vi "test_read-nmea-data2.vi"() -> ()   [LabVIEW 2019] (continued)
23,06,64,050,35,6*6E\n\t\n15:13:22.46\tF9P\t$GPGSV,3,2,09,09,45,074,31,12,23,276,26,17,33,154,28,19,52,157,,6*67\n\t\n15:13:22.48\tF9P\t$GPGSV,3,3,09,25,12,306,,6*5B\n\t\n15:13:22.50\tF9P\t$GLGSV,2,1,08,69,11,031,36,70,70,038,25,71,53,206,41,72,05,210,19,1*7D\n\t\n15:13:22.52\tF9P\t$GLGSV,2,2,08,77,01,325,,84,19,123,11,85,70,070,32,86,37,330,,1*77\n\t\n15:13:22.54\tF9P\t$GLGSV,2,1,08,69,11,031,26,70,70,038,,71,53,206,27,72,05,210,,3*71\n\t\n15:13:22.56\tF9P\t$GLGSV,2,2,08,77,01,325,,84,19,123,17,85,70,070,24,86,37,330,,3*74\n\t\n15:13:22.58\tF9P\t$GAGSV,2,1,08,02,08,297,11,04,66,116,30,09,32,193,35,11,72,359,26,7*74\n\t\n15:13:22.60\tF9P\t$GAGSV,2,2,08,12,40,103,32,19,26,045,18,25,09,249,,36,26,308,21,7*73\n\t\n15:13:22.62\tF9P\t$GAGSV,2,1,08,02,08,297,,04,66,116,,09,32,193,,11,72,359,,2*70\n\t\n15:13:22.64\tF9P\t$GAGSV,2,2,08,12,40,103,,19,26,045,,25,09,249,,36,26,308,,2*7D\n\t\n15:13:22.66\tF9P\t$GBGSV,1,1,04,11,49,132,29,14,87,114,27,28,,,29,33,61,220,32,1*48\n\t\n15:13:22.68\tF9P\t$GBGSV,1,1,04,11,49,132,34,14,87,114,,25,,,05,33,61,220,,3*41\n\t\n15:13:22.70\tF9P\t$GNGLL,3723.55902,N,12656.98306,E,061324.00,A,A*79\n\t\n15:13:22.72\tF9P\t\t\n15:13:22.74\tF9P\t\t\n15:13:22.76\tF9P\t\t\n15:13:22.78\tF9P\t\t\n15:13:22.80\tF9P\t\t\n15:13:22.82\tF9P\t\t\n15:13:22.84\tF9P\t\t\n15:13:22.86\tF9P\t\t\n15:13:22.88\tF9P\t\t\n15:13:22.90\tF9P\t\t\n15:13:22.92\tF9P\t\t\n15:13:22.94\tF9P\t\t\n15:13:22.96\tF9P\t\t\n15:13:22.98\tF9P\t\t\n15:13:23.00\tF9P\t\t\n15:13:23.02\tF9P\t\t\n15:13:23.04\tF9P\t\t\n15:13:23.06\tF9P\t\t\n15:13:23.08\tF9P\t\t\n15:13:23.10\tF9P\t\t\n15:13:23.12\tF9P\t\t\n15:13:23.14\tF9P\t\t\n15:13:23.16\tF9P\t\t\n15:13:23.18\tF9P\t\t\n15:13:23.20\tF9P\t\t\n15:13:23.22\tF9P\t\t\n15:13:23.24\tF9P\t$GNRMC,061325.00,A,3723.55967,N,12656.98378,E,2.656,30.39,250720,,,A,V*33\n\t\n15:13:23.26\tF9P\t$GNVTG,30.39,T,,M,2.656,N,4.919,K,A*18\n\t\n15:13:23.28\tF9P\t$GNGGA,061325.00,3723.55967,N,12656.98378,E,1,12,0.68,50.1,M,18.5,M,,*72\n\t\n15:13:23.30\tF9P\t$GNGSA,A,3,12,06,19,05,17,09,04,02,,,,,1.20,0.68,0.99,1*0D\n\t\n15:13:23.32\tF9P\t$GNGSA,A,3,85,70,71,84,,,,,,,,,1.20,0.68,0.99,2*0F\n\t\n15:13:23.34\tF9P\t$GNGSA,A,3,36,19,11,04,09,12,,,,,,,1.20,0.68,0.99,3*0D\n\t\n15:13:23.36\tF9P\t$GNGSA,A,3,14,11,33,,,,,,,,,,1.20,0.68,0.99,4*0C\n\t\n15:13:23.38\tF9P\t$GPGSV,3,1,09,02,55,320,30,04,17,043,23,05,38,248,37,06,64,050,30,1*6D\n\t\n15:13:23.40\tF9P\t$GPGSV,3,2,09,09,45,074,33,12,23,276,39,17,33,154,37,19,52,157,31,1*60\n\t\n15:13:23.42\tF9P\t$GPGSV,3,3,09,25,12,306,21,1*5F\n\t\n15:13:23.44\tF9P\t$GPGSV,3,1,09,02,55,320,,04,17,043,16,05,38,248,22,06,64,050,35,6*6E\n\t\n15:13:23.46\tF9P\t$GPGSV,3,2,09,09,45,074,33,12,23,276,26,17,33,154,27,19,52,157,,6*6A\n\t\n15:13:23.48\tF9P\t$GPGSV,3,3,09,25,12,306,,6*5B\n\t\n15:13:23.50\tF9P\t$GLGSV,2,1,08,69,11,031,31,70,70,038,25,71,53,206,33,72,05,210,21,1*74\n\t\n15:13:23.52\tF9P\t$GLGSV,2,2,08,77,01,325,,84,19,123,14,85,70,070,39,86,37,330,,1*79\n\t\n15:13:23.54\tF9P\t$GLGSV,2,1,08,69,11,031,31,70,70,038,,71,53,206,25,72,05,210,,3*75\n\t\n15:13:23.56\tF9P\t$GLGSV,2,2,08,77,01,325,,84,19,123,16,85,70,070,25,86,37,330,,3*74\n\t\n15:13:23.58\tF9P\t$GAGSV,2,1,08,02,08,297,08,04,66,116,29,09,32,193,37,11,72,359,27,7*77\n\t\n15:13:23.60\tF9P\t$GAGSV,2,2,08,12,40,103,27,19,26,045,18,25,09,249,,36,26,308,20,7*76\n\t\n15:13:23.62\tF9P\t$GAGSV,2,1,08,02,08,297,,04,66,116,,09,32,193,,11,72,359,,2*70\n\t\n15:13:23.64\tF9P\t$GAGSV,2,2,08,12,40,103,,19,26,045,,25,09,249,,36,26,308,,2*7D\n\t\n15:13:23.66\tF9P\t$GBGSV,1,1,04,11,49,132,33,14,87,114,28,28,,,29,33,61,220,27,1*48\n\t\n15:13:23.68\tF9P\t$GBGSV,1,1,03,11,49,132,30,14,87,114,,33,61,220,,3*40\n\t\n15:13:23.70\tF9P\t$GNGLL,3723.55967,N,12656.98378,E,061325.00,A,A*72\n\t\n15:13:23.72\tF9P\t\t\n15:13:23.74\tF9P\t\t\n15:13:23.76\tF9P\t\t\n15:13:23.78\tF9P\t\t\n15:13:23.80\tF9P\t\t\n15:13:23.82\tF9P\t\t\n15:13:23.84\tF9P\t\t\n15:13:23.86\tF9P\t\t\n15:13:23.88\tF9P\t\t\n15:13:23.90\tF9P\t\t\n15:13:23.92\tF9P\t\t\n15:13:23.94\tF9P\t\t\n15:13:23.96\tF9P\t\t\n15:13:23.98\tF9P\t\t\n15:13:24.00\tF9P\t\t\n15:13:24.02\tF9P\t\t\n15:13:24.04\tF9P\t\t\n15:13:24.06\tF9P\t\t\n15:13:24.08\tF9P\t\t\n15:13:24.10\tF9P\t\t\n15:13:24.12\tF9P\t\t\n15:13:24.14\tF9P\t\t\n15:13:24.16\tF9P\t\t\n15:13:24.18\tF9P\t\t\n15:13:24.20\tF9P\t\t\n15:13:24.22\tF9P\t\t\n15:13:24.24\tF9P\t$GNRMC,061326.00,A,3723.56015,N,12656.98454,E,2.542,31.14,250720,,,A,V*3E\n\t\n15:13:24.26\tF9P\t$GNVTG,31.14,T,,M,2.542,N,4.708,K,A*1E\n\t\n15:13:24.28\tF9P\t$GNGGA,061326.00,3723.56015,N,12656.98454,E,1,12,0.71,50.6,M,18.5,M,,*78\n\t\n15:13:24.30\tF9P\t$GNGSA,A,3,12,06,19,05,17,09,04,02,,,,,1.26,0.71,1.04,1*06\n\t\n15:13:24.32\tF9P\t$GNGSA,A,3,85,70,71,84,,,,,,,,,1.26,0.71,1.04,2*04\n\t\n15:13:24.34\tF9P\t$GNGSA,A,3,36,19,11,04,09,12,,,,,,,1.26,0.71,1.04,3*06\n\t\n15:13:24.36\tF9P\t$GNGSA,A,3,14,11,33,,,,,,,,,,1.26,0.71,1.04,4*07\n\t\n15:13:24.38\tF9P\t$GPGSV,3,1,09,02,55,320,35,04,17,043,23,05,38,248,26,06,64,050,30,1*68\n\t\n15:13:24.40\tF9P\t$GPGSV,3,2,09,09,45,074,36,12,23,276,42,17,33,154,30,19,52,157,29,1*67\n\t\n15:13:24.42\tF9P\t$GPGSV,3,3,09,25,12,306,20,1*5E\n\t\n15:13:24.44\tF9P\t$GPGSV,3,1,09,02,55,320,,04,17,043,15,05,38,248,18,06,64,050,31,6*60\n\t\n15:13:24.46\tF9P\t$GPGSV,3,2,09,09,45,074,33,12,23,276,26,17,33,154,24,19,52,157,,6*69\n\t\n15:13:24.48\tF9P\t$GPGSV,3,3,09,25,12,306,,6*5B\n\t\n15:13:24.50\tF9P\t$GLGSV,2,1,08,69,11,031,33,70,70,038,26,71,53,206,33,72,05,210,21,1*75\n\t\n15:13:24.52\tF9P\t$GLGSV,2,2,08,77,01,325,,84,19,123,08,85,70,070,31,86,37,330,,1*7C\n\t\n15:13:24.54\tF9P\t$GLGSV,2,1,08,69,11,031,31,70,70,038,,71,53,206,24,72,05,210,,3*74\n\t\n15:13:24.56\tF9P\t$GLGSV,2,2,08,77,01,325,,84,19,123,16,85,70,070,27,86,37,330,,3*76\n\t\n15:13:24.58\tF9P\t$GAGSV,2,1,08,02,08,297,11,04,66,116,33,09,32,193,39,11,72,359,27,7*7A\n\t\n15:13:24.60\tF9P\t$GAGSV,2,2,08,12,40,103,32,19,26,045,18,25,09,249,,36,26,308,21,7*73\n\t\n15:13:24.62\tF9P\t$GAGSV,2,1,08,02,08,297,,04,66,116,,09,32,193,,11,72,359,,2*70\n\t\n15:13:24.64\tF9P\t$GAGSV,2,2,08,12,40,103,,19,26,045,,25,09,249,,36,26,308,,2*7D\n\t\n15:13:24.66\tF9P\t$GBGSV,1,1,04,11,49,132,27,14,87,114,33,28,,,33,33,61,220,32,1*48\n\t\n15:13:24.68\tF9P\t$GBGSV,1,1,03,11,49,132,29,14,87,114,,33,61,220,,3*48\n\t\n15:13:24.70\tF9P\t$GNGLL,3723.56015,N,12656.98454,E,061326.00,A,A*77\n\t\n15:13:24.72\tF9P\t\t\n15:13:24.74\tF9P\t\t\n15:13:24.76\tF9P\t\t\n15:13:24.78\tF9P\t\t\n15:13:24.80\tF9P\t\t\n15:13:24.82\tF9P\t\t\n15:13:24.84\tF9P\t\t\n15:13:24.86\tF9P\t\t\n15:13:24.88\tF9P\t\t\n15:13:24.90\tF9P\t\t\n15:13:24.92\tF9P\t\t\n15:13:24.94\tF9P\t\t\n15:13:24.96\tF9P\t\t\n15:13:24.98\tF9P\t\t\n15:13:25.00\tF9P\t\t\n15:13:25.02\tF9P\t\t\n15:13:25.04\tF9P\t\t\n15:13:25.06\tF9P\t\t\n15:13:25.08\tF9P\t\t\n15:13:25.10\tF9P\t\t\n15:13:25.12\tF9P\t\t\n15:13:25.14\tF9P\t\t\n15:13:25.16\tF9P\t\t\n15:13:25.18\tF9P\t\t\n15:13:25.20\tF9P\t\t\n15:13:25.22\tF9P\t\t\n15:13:25.24\tF9P\t$GNRMC,061327.00,A,3723.56072,N,12656.98531,E,2.555,25.42,250720,,,A,V*3C\n\t\n15:13:25.26\tF9P\t$GNVTG,25.42,T,,M,2.555,N,4.733,K,A*16\n\t\n15:13:25.28\tF9P\t$GNGGA,061327.00,3723.56072,N,12656.98531,E,1,12,0.71,50.7,M,18.5,M,,*7B\n\t\n15:13:25.30\tF9P\t$GNGSA,A,3,12,06,19,05,17,09,04,02,,,,,1.26,0.71,1.04,1*06\n\t\n15:13:25.32\tF9P\t$GNGSA,A,3,85,70,71,84,,,,,,,,,1.26,0.71,1.04,2*04\n\t\n15:13:25.34\tF9P\t$GNGSA,A,3,36,19,11,04,09,12,,,,,,,1.26,0.71,1.04,3*06\n\t\n15:13:25.36\tF9P\t$GNGSA,A,3,14,11,33,,,,,,,,,,1.26,0.71,1.04,4*07\n\t\n15:13:25.38\tF9P\t$GPGSV,3,1,09,02,55,320,28,04,17,043,24,05,38,248,40,06,64,050,33,1*60\n\t\n15:13:25.40\tF9P\t$GPGSV,3,2,09,09,44,073,28,12,23,276,46,17,33,154,38,19,52,157,31,1*6B\n\t\n15:13:25.42\tF9P\t$GPGSV,3,3,09,25,12,306,19,1*54\n\t\n15:13:25.44\tF9P\t$GPGSV,3,1,09,02,55,320,,04,17,043,15,05,38,248,17,06,64,050,32,6*6C\n\t\n15:13:25.46\tF9P\t$GPGSV,3,2,09,09,44,073,35,12,23,276,25,17,33,154,25,19,52,157,,6*6B\n\t\n15:13:25.48\tF9P\t$GPGSV,3,3,09,25,12,306,,6*5B\n\t\n15:13:25.50\tF9P\t$GLGSV,2,1,08,69,11,031,33,70,70,038,26,71,53,206,34,72,05,210,20,1*73\n\t\n15:13:25.52\tF9P\t$GLGSV,2,2,08,77,01,325,,84,19,123,11,85,70,070,32,86,37,330,,1*77\n\t\n15:13:25.54\tF9P\t$GLGSV,2,1,08,69,11,031,23,70,70,038,,71,53,206,25,72,05,210,,3*76\n\t\n15:13:25.56\tF9P\t$GLGSV,2,2,08,77,01,325,,84,19,123,18,85,70,070,26,86,37,330,,3*79\n\t\n15:13:25.58\tF9P\t$GAGSV,2,1,08,02,08,297,10,04,66,116,28,09,32,193,38,11,72,359,27,7*70\n\t\n15:13:25.60\tF9P\t$GAGSV,2,2,08,12,40,103,28,19,26,045,17,25,09,249,,36,26,308,20,7*76\n\t\n15:13:25.62\tF9P\t$GAGSV,2,1,08,02,08,297,,04,66,116,,09,32,193,,11,72,359,,2*70\n\t\n15:13:25.64\tF9P\t$GAGSV,2,2,08,12,40,103,,19,26,045,,25,09,249,,36,26,308,,2*7D\n\t\n15:13:25.66\tF9P\t$GBGSV,1,1,04,11,49,132,28,14,87,114,31,28,,,32,33,61,220,28,1*4F\n\t\n15:13:25.68\tF9P\t$GBGSV,1,1,03,11,49,132,32,14,87,114,,33,61,220,,3*42\n\t\n15:13:25.70\tF9P\t$GNGLL,3723.56072,N,12656.98531,E,061327.00,A,A*75\n\t\n15:13:25.72\tF9P\t\t\n15:13:25.74\tF9P\t\t\n15:13:25.76\tF9P\t\t\n15:13:25.78\tF9P\t\t\n15:13:25.80\tF9P\t\t\n15:13:25.82\tF9P\t\t\n15:13:25.84\tF9P\t\t\n15:13:25.86\tF9P\t\t\n15:13:25.88\tF9P\t\t\n15:13:25.90\tF9P\t\t\n15:13:25.92\tF9P\t\t\n15:13:25.94\tF9P\t\t\n15:13:25.96\tF9P\t\t\n15:13:25.98\tF9P\t\t\n15:13:26.00\tF9P\t\t\n15:13:26.02\tF9P\t\t\n15:13:26.04\tF9P\t\t\n15:13:26.06\tF9P\t\t\n15:13:26.08\tF9P\t\t\n15:13:26.10\tF9P\t\t\n15:13:26.12\tF9P\t\t\n15:13:26.14\tF9P\t\t\n15:13:26.16\tF9P\t\t\n15:13:26.18\tF9P\t\t\n15:13:26.20\tF9P\t\t\n15:13:26.22\tF9P\t\t\n15:13:26.24\tF9P\t$GNRMC,061328.00,A,3723.56131,N,12656.98590,E,2.306,24.51,250720,,,A,V*3D\n\t\n15:13:26.26\tF9P\t$GNVTG,24.51,T,,M,2.306,N,4.270,K,A*17\n\t\n15:13:26.28\tF9P\t$GNGGA,061328.00,3723.56131,N,12656.98590,E,1,12,0.84,50.2,M,18.5,M,,*76\n\t\n15:13:26.30\tF9P\t$GNGSA,A,3,12,06,19,05,17,09,04,02,,,,,1.55,0.84,1.30,1*0F\n\t\n15:13:26.32\tF9P\t$GNGSA,A,3,85,70,71,84,,,,,,,,,1.55,0.84,1.30,2*0D\n\t\n15:13:26.34\tF9P\t$GNGSA,A,3,36,19,11,04,09,12,,,,,,,1.55,0.84,1.30,3*0F\n\t\n15:13:26.36\tF9P\t$GNGSA,A,3,14,11,33,,,,,,,,,,1.55,0.84,1.30,4*0E\n\t\n15:13:26.38\tF9P\t$GPGSV,3,1,09,02,55,320,32,04,17,043,22,05,38,248,34,06,64,050,30,1*6D\n\t\n15:13:26.40\tF9P\t$GPGSV,3,2,09,09,44,073,28,12,23,276,48,17,33,154,42,19,52,157,28,1*60\n\t\n15:13:26.42\tF9P\t$GPGSV,3,3,09,25,12,306,20,1*5E\n\t\n15:13:26.44\tF9P\t$GPGSV,3,1,09,02,55,320,,04,17,043,16,05,38,248,20,06,64,050,31,6*68\n\t\n15:13:26.46\tF9P\t$GPGSV,3,2,09,09,44,073,35,12,23,276,24,17,33,154,28,19,52,157,,6*67\n\t\n15:13:26.48\tF9P\t$GPGSV,3,3,09,25,12,306,,6*5B\n\t\n15:13:26.50\tF9P\t$GLGSV,2,1,08,69,11,031,33,70,70,038,23,71,53,206,39,72,05,210,20,1*7B\n\t\n15:13:26.52\tF9P\t$GLGSV,2,2,08,77,01,325,,84,19,123,17,85,70,070,32,86,37,330,,1*71\n\t\n15:13:26.54\tF9P\t$GLGSV,2,1,08,69,11,031,25,70,70,038,,71,53,206,26,72,05,210,,3*73\n\t\n15:13:26.56\tF9P\t$GLGSV,2,2,08,77,01,325,,84,19,123,20,85,70,070,25,86,37,330,,3*71\n\t\n15:13:26.58\tF9P\t$GAGSV,2,1,08,02,08,297,09,04,66,116,28,09,32,193,43,11,72,359,27,7*74\n\t\n15:13:26.60\tF9P\t$GAGSV,2,2,08,12,40,103,27,19,26,045,16,25,09,249,,36,26,308,19,7*72\n\t\n15:13:26.62\tF9P\t$GAGSV,2,1,08,02,08,297,,04,66,116,,09,32,193,,11,72,359,,2*70\n\t\n15:13:26.64\tF9P\t$GAGSV,2,2,08,12,40,103,,19,26,045,,25,09,249,,36,26,308,,2*7D\n\t\n15:13:26.66\tF9P\t$GBGSV,1,1,04,11,49,132,28,14,87,114,32,28,,,32,33,61,220,37,1*42\n\t\n15:13:26.68\tF9P\t$GBGSV,1,1,03,11,49,132,32,14,87,114,,33,61,220,,3*42\n\t\n15:13:26.70\tF9P\t$GNGLL,3723.56131,N,12656.98590,E,061328.00,A,A*77\n\t\n15:13:26.72\tF9P\t\t\n15:13:26.74\tF9P\t\t\n15:13:26.76\tF9P\t\t\n15:13:26.78\tF9P\t\t\n15:13:26.80\tF9P\t\t\n15:13:26.82\tF9P\t\t\n15:13:26.84\tF9P\t\t\n15:13:26.86\tF9P\t\t\n15:13:26.88\tF9P\t\t\n15:13:26.90\tF9P\t\t\n15:13:26.92\tF9P\t\t\n15:13:26.94\tF9P\t\t\n15:13:26.96\tF9P\t\t\n15:13:26.98\tF9P\t\t\n15:13:27.00\tF9P\t\t\n15:13:27.02\tF9P\t\t\n15:13:27.04\tF9P\t\t\n15:13:27.06\tF9P\t\t\n15:13:27.08\tF9P\t\t\n15:13:27.10\tF9P\t\t\n15:13:27.12\tF9P\t\t\n15:13:27.14\tF9P\t\t\n15:13:27.16\tF9P\t\t\n15:13:27.18\tF9P\t\t\n15:13:27.20\tF9P\t\t\n15:13:27.22\tF9P\t\t\n15:13:27.24\tF9P\t$GNRMC,061329.00,A,3723.56180,N,12656.98626,E,2.237,8.16,250720,,,A,V*06\n\t\n15:13:27.26\tF9P\t$GNVTG,8.16,T,,M,2.237,N,4.143,K,A*2A\n\t\n15:13:27.28\tF9P\t$GNGGA,061329.00,3723.56180,N,12656.98626,E,1,12,0.82,50.4,M,18.5,M,,*73\n\t\n15:13:27.30\tF9P\t$GNGSA,A,3,12,06,19,05,17,09,04,02,,,,,1.52,0.82,1.28,1*07\n\t\n15:13:27.32\tF9P\t$GNGSA,A,3,85,70,71,84,,,,,,,,,1.52,0.82,1.28,2*05\n\t\n15:13:27.34\tF9P\t$GNGSA,A,3,36,19,11,04,09,12,,,,,,,1.52,0.82,1.28,3*07\n\t\n15:13:27.36\tF9P\t$GNGSA,A,3,14,11,33,,,,,,,,,,1.52,0.82,1.28,4*06\n\t\n15:13:27.38\tF9P\t$GPGSV,3,1,09,02,55,320,26,04,17,043,22,05,38,248,46,06,64,050,32,1*6F\n\t\n15:13:27.40\tF9P\t$GPGSV,3,2,09,09,44,073,29,12,23,276,45,17,33,154,44,19,52,157,36,1*65\n\t\n15:13:27.42\tF9P\t$GPGSV,3,3,09,25,12,306,22,1*5C\n\t\n15:13:27.44\tF9P\t$GPGSV,3,1,09,02,55,320,,04,17,043,16,05,38,248,23,06,64,050,26,6*6D\n\t\n15:13:27.46\tF9P\t$GPGSV,3,2,09,09,44,073,27,12,23,276,35,17,33,154,31,19,52,157,,6*6C\n\t\n15:13:27.48\tF9P\t$GPGSV,3,3,09,25,12,306,,6*5B\n\t\n15:13:27.50\tF9P\t$GLGSV,2,1,08,69,11,031,31,70,70,038,23,71,53,206,36,72,05,210,19,1*7C\n\t\n15:13:27.52\tF9P\t$GLGSV,2,2,08,77,01,325,,84,19,123,16,85,70,070,33,86,37,330,,1*71\n\t\n15:13:27.54\tF9P\t$GLGSV,2,1,08,69,11,031,25,70,70,038,,71,53,206,26,72,05,210,,3*73\n\t\n15:13:27.56\tF9P\t$GLGSV,2,2,08,77,01,325,,84,19,123,21,85,70,070,25,86,37,330,,3*70\n\t\n15:13:27.58\tF9P\t$GAGSV,2,1,08,02,08,297,10,04,66,116,28,09,32,193,44,11,72,359,19,7*76\n\t\n15:13:27.60\tF9P\t$GAGSV,2,2,08,12,40,103,27,19,26,045,15,25,09,249,,36,26,308,18,7*70\n\t\n15:13:27.62\tF9P\t$GAGSV,2,1,08,02,08,297,,04,66,116,,09,32,193,39,11,72,359,,2*7A\n\t\n15:13:27.64\tF9P\t$GAGSV,2,2,08,12,40,103,,19,26,045,,25,09,249,,36,26,308,,2*7D\n\t\n15:13:27.66\tF9P\t$GBGSV,1,1,04,11,49,132,33,14,87,114,32,28,,,29,33,61,220,31,1*44\n\t\n15:13:27.68\tF9P\t$GBGSV,1,1,03,11,49,132,32,14,87,114,29,33,61,220,,3*49\n\t\n15:13:27.70\tF9P\t$GNGLL,3723.56180,N,12656.98626,E,061329.00,A,A*72\n\t\n15:13:27.72\tF9P\t\t\n15:13:27.74\tF9P\t\t\n15:13:27.76\tF9P\t\t\n15:13:27.78\tF9P\t\t\n15:13:27.80\tF9P\t\t\n15:13:27.82\tF9P\t\t\n15:13:27.84\tF9P\t\t\n15:13:27.86\tF9P\t\t\n15:13:27.88\tF9P\t\t\n15:13:27.90\tF9P\t\t\n15:13:27.92\tF9P\t\t\n15:13:27.94\tF9P\t\t\n15:13:27.96\tF9P\t\t\n15:13:27.98\tF9P\t\t\n15:13:28.00\tF9P\t\t\n15:13:28.02\tF9P\t\t\n15:13:28.04\tF9P\t\t\n15:13:28.06\tF9P\t\t\n15:13:28.08\tF9P\t\t\n15:13:28.10\tF9P\t\t\n15:13:28.12\tF9P\t\t\n15:13:28.14\tF9P\t\t\n15:13:28.16\tF9P\t\t\n15:13:28.18\tF9P\t\t\n15:13:28.20\tF9P\t\t\n15:13:28.22\tF9P\t\t\n15:13:28.24\tF9P\t$GNRMC,061330.00,A,3723.56218,N,12656.98657,E,2.150,3.44,250720,,,A,V*04\n\t\n15:13:28.26\tF9P\t$GNVTG,3.44,T,,M,2.150,N,3.982,K,A*26\n\t\n15:13:28.28\tF9P\t$GNGGA,061330.00,3723.56218,N,12656.98657,E,1,12,0.71,51.2,M,18.5,M,,*74\n\t\n15:13:28.30\tF9P\t$GNGSA,A,3,12,06,19,05,17,09,04,02,,,,,1.26,0.71,1.04,1*06\n\t\n15:13:28.32\tF9P\t$GNGSA,A,3,85,70,71,84,,,,,,,,,1.26,0.71,1.04,2*04\n\t\n15:13:28.34\tF9P\t$GNGSA,A,3,36,19,11,04,09,12,,,,,,,1.26,0.71,1.04,3*06\n\t\n15:13:28.36\tF9P\t$GNGSA,A,3,14,11,33,,,,,,,,,,1.26,0.71,1.04,4*07\n\t\n15:13:28.38\tF9P\t$GPGSV,3,1,09,02,55,320,25,04,17,043,22,05,38,248,26,06,64,050,26,1*6F\n\t\n15:13:28.40\tF9P\t$GPGSV,3,2,09,09,44,073,33,12,23,276,36,17,33,154,43,19,52,157,27,1*6D\n\t\n15:13:28.42\tF9P\t$GPGSV,3,3,09,25,12,306,23,1*5D\n\t\n15:13:28.44\tF9P\t$GPGSV,3,1,09,02,55,320,,04,17,043,16,05,38,248,21,06,64,050,26,6*6F\n\t\n15:13:28.46\tF9P\t$GPGSV,3,2,09,09,44,073,27,12,23,276,32,17,33,154,26,19,52,157,,6*6D\n\t\n15:13:28.48\tF9P\t$GPGSV,3,3,09,25,12,306,,6*5B\n\t\n15:13:28.50\tF9P\t$GLGSV,2,1,08,69,11,031,35,70,70,038,23,71,53,206,32,72,05,210,19,1*7C\n\t\n15:13:28.52\tF9P\t$GLGSV,2,2,08,77,01,325,,84,19,123,20,85,70,070,35,86,37,330,,1*72\n\t\n15:13:28.54\tF9P\t$GLGSV,2,1,08,69,11,031,26,70,70,038,,71,53,206,25,72,05,210,,3*73\n\t\n15:13:28.56\tF9P\t$GLGSV,2,2,08,77,01,325,,84,19,123,23,85,70,070,25,86,37,330,,3*72\n\t\n15:13:28.58\tF9P\t$GAGSV,2,1,08,02,08,297,12,04,66,116,27,09,32,193,35,11,72,359,20,7*77\n\t\n15:13:28.60\tF9P\t$GAGSV,2,2,08,12,40,103,35,19,26,045,15,25,09,249,,36,26,308,17,7*7C\n\t\n15:13:28.62\tF9P\t$GAGSV,2,1,08,02,08,297,,04,66,116,,09,32,193,30,11,72,359,,2*73\n\t\n15:13:28.64\tF9P\t$GAGSV,2,2,08,12,40,103,,19,26,045,,25,09,249,,36,26,308,,2*7D\n\t\n15:13:28.66\tF9P\t$GBGSV,1,1,04,11,49,132,30,14,87,114,26,28,,,24,33,61,220,28,1*47\n\t\n15:13:28.68\tF9P\t$GBGSV,1,1,03,11,49,132,31,14,87,114,21,33,61,220,,3*42\n\t\n15:13:28.70\tF9P\t$GNGLL,3723.56218,N,12656.98657,E,061330.00,A,A*7E\n\t\n15:13:28.72\tF9P\t\t\n15:13:28.74\tF9P\t\t\n15:13:28.76\tF9P\t\t\n15:13:28.78\tF9P\t\t\n15:13:28.80\tF9P\t\t\n15:13:28.82\tF9P\t\t\n15:13:28.84\tF9P\t\t\n15:13:28.86\tF9P\t\t\n15:13:28.88\tF9P\t\t\n15:13:28.90\tF9P\t\t\n15:13:28.92\tF9P\t\t\n15:13:28.94\tF9P\t\t\n15:13:28.96\tF9P\t\t\n15:13:28.98\tF9P\t\t\n15:13:29.00\tF9P\t\t\n15:13:29.02\tF9P\t\t\n15:13:29.04\tF9P\t\t\n15:13:29.06\tF9P\t\t\n15:13:29.08\tF9P\t\t\n15:13:29.10\tF9P\t\t\n15:13:29.12\tF9P\t\t\n15:13:29.14\tF9P\t\t\n15:13:29.16\tF9P\t\t\n15:13:29.18\tF9P\t\t\n15:13:29.20\tF9P\t\t\n15:13:29.22\tF9P\t\t\n15:13:29.24\tF9P\t$GNRMC,061331.00,A,3723.56311,N,12656.98715,E,3.075,17.29,250720,,,A,V*33\n\t\n15:13:29.26\tF9P\t$GNVTG,17.29,T,,M,3.075,N,5.695,K,A*10\n\t\n15:13:29.28\tF9P\t$GNGGA,061331.00,3723.56311,N,12656.98715,E,1,12,0.95,49.1,M,18.5,M,,*7A\n\t\n15:13:29.30\tF9P\t$GNGSA,A,3,12,06,19,05,17,09,04,02,,,,,1.88,0.95,1.62,1*08\n\t\n15:13:29.32\tF9P\t$GNGSA,A,3,85,70,71,84,,,,,,,,,1.88,0.95,1.62,2*0A\n\t\n15:13:29.34\tF9P\t$GNGSA,A,3,36,19,11,04,09,12,,,,,,,1.88,0.95,1.62,3*08\n\t\n15:13:29.36\tF9P\t$GNGSA,A,3,14,11,33,,,,,,,,,,1.88,0.95,1.62,4*09\n\t\n15:13:29.38\tF9P\t$GPGSV,3,1,09,02,55,320,26,04,17,043,23,05,38,248,26,06,64,050,28,1*63\n\t\n15:13:29.40\tF9P\t$GPGSV,3,2,09,09,44,073,30,12,23,276,31,17,33,154,45,19,52,157,33,1*6A\n\t\n15:13:29.42\tF9P\t$GPGSV,3,3,09,25,12,306,25,1*5B\n\t\n15:13:29.44\tF9P\t$GPGSV,3,1,09,02,55,320,,04,17,043,16,05,38,248,18,06,64,050,26,6*65\n\t\n15:13:29.46\tF9P\t$GPGSV,3,2,09,09,44,073,32,12,23,276,26,17,33,154,26,19,52,157,,6*6C\n\t\n15:13:29.48\tF9P\t$GPGSV,3,3,09,25,12,306,,6*5B\n\t\n15:13:29.50\tF9P\t$GLGSV,2,1,08,69,11,031,25,70,70,038,22,71,53,206,27,72,05,210,19,1*78\n\t\n15:13:29.52\tF9P\t$GLGSV,2,2,08,77,01,325,,84,19,123,21,85,70,070,27,86,37,330,,1*70\n\t\n15:13:29.54\tF9P\t$GLGSV,2,1,08,69,11,031,24,70,70,038,,71,53,206,22,72,05,210,,3*76\n\t\n15:13:29.56\tF9P\t$GLGSV,2,2,08,77,01,325,,84,19,123,31,85,70,070,24,86,37,330,,3*70\n\t\n15:13:29.58\tF9P\t$GAGSV,2,1,08,02,08,297,09,04,66,116,26,09,32,193,26,11,72,359,23,7*7D\n\t\n15:13:29.60\tF9P\t$GAGSV,2,2,08,12,40,103,33,19,26,045,15,25,09,249,21,36,26,308,16,7*78\n\t\n15:13:29.62\tF9P\t$GAGSV,2,1,08,02,08,297,,04,66,116,,09,32,193,,11,72,359,,2*70\n\t\n15:13:29.64\tF9P\t$GAGSV,2,2,08,12,40,103,,19,26,045,,25,09,249,,36,26,308,,2*7D\n\t\n15:13:29.66\tF9P\t$GBGSV,1,1,04,11,49,132,34,14,87,114,26,28,,,29,33,61,220,27,1*41\n\t\n15:13:29.68\tF9P\t$GBGSV,1,1,03,11,49,132,34,14,87,114,22,33,61,220,,3*44\n\t\n15:13:29.70\tF9P\t$GNGLL,3723.56311,N,12656.98715,E,061331.00,A,A*70\n\t\n15:13:29.72\tF9P\t\t\n15:13:29.74\tF9P\t\t\n15:13:29.76\tF9P\t\t\n15:13:29.78\tF9P\t\t\n15:13:29.80\tF9P\t\t\n15:13:29.82\tF9P\t\t\n15:13:29.84\tF9P\t\t\n15:13:29.86\tF9P\t\t\n15:13:29.88\tF9P\t\t\n15:13:29.90\tF9P\t\t\n15:13:29.92\tF9P\t\t\n15:13:29.94\tF9P\t\t\n15:13:29.96\tF9P\t\t\n15:13:29.98\tF9P\t\t\n15:13:30.00\tF9P\t\t\n15:13:30.02\tF9P\t\t\n15:13:30.04\tF9P\t\t\n15:13:30.06\tF9P\t\t\n15:13:30.08\tF9P\t\t\n15:13:30.10\tF9P\t\t\n15:13:30.12\tF9P\t\t\n15:13:30.14\tF9P\t\t\n15:13:30.16\tF9P\t\t\n15:13:30.18\tF9P\t\t\n15:13:30.20\tF9P\t\t\n15:13:30.22\tF9P\t$GNRMC,061332.00,A,3723.56358,N,12656.98749,E,2.299,14.12,250720,,,A,V*3E\n\t\n15:13:30.24\tF9P\t$GNVTG,14.12,T,,M,2.299,N,4.258,K,A*1E\n\t\n15:13:30.26\tF9P\t$GNGGA,061332.00,3723.56358,N,12656.98749,E,1,12,0.95,49.9,M,18.5,M,,*75\n\t\n15:13:30.28\tF9P\t$GNGSA,
